vi "HandleStopSync.vi"(8 "error in (no error)":errorcluster, 11 "S4GUI in":refnum<class "S4GUI.lvclass">) -> (0 "error out":errorcluster, 3 "S4GUI out":refnum<class "S4GUI.lvclass">)   [LabVIEW 2018, in "S4GUI.lvclass"]
uses:
  S4GUI.lvclass
  S4GUI.lvclass/S4GUI.ctl
  Instrument/Instrument.lvclass/Instrument.ctl
  Instrument/Instrument.lvclass
  Device/Optics/Opt_Selector/Opt_Selector.lvclass
  Acquisition/Acquisition.lvclass
  StateMachine/State Machine.lvclass
  Channel/Channel.lvclass
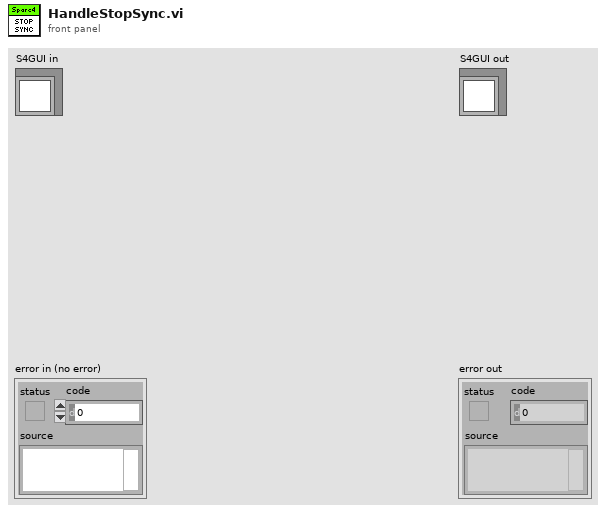
[diagram p1: front panel]
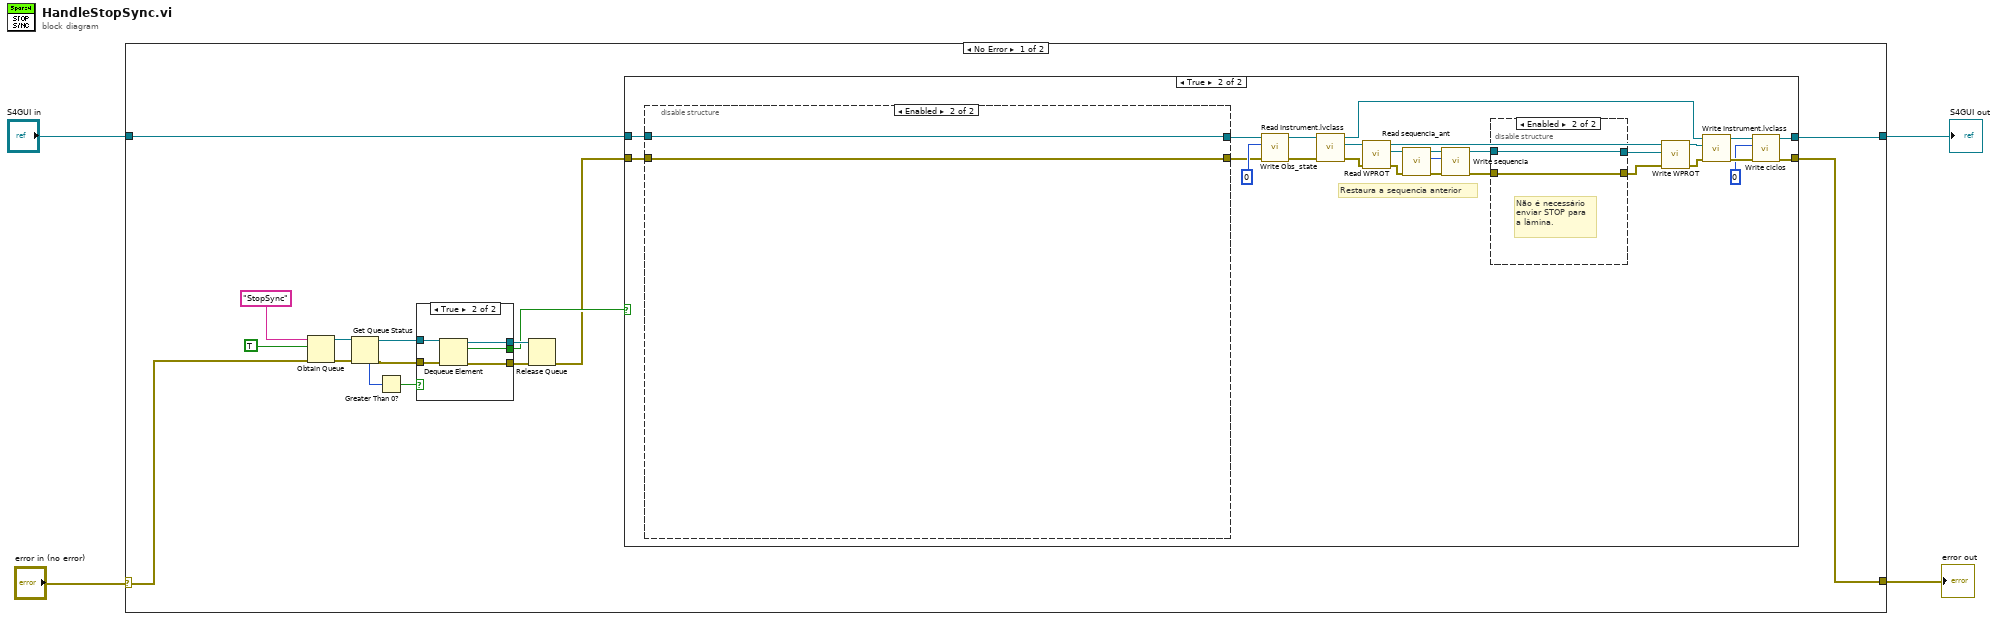
[diagram p0: block diagram]
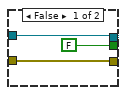
[diagram p2: hidden frame]
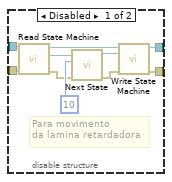
[diagram p4: hidden frame]
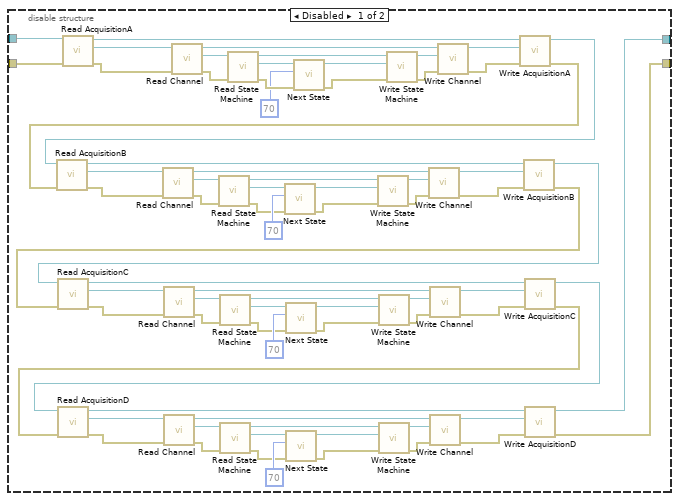
[diagram p5: hidden frame]
diagram:
  n1 = case shown="No Error" "error in (no error)" {
    selector: "error in (no error)" -> [w7 w147]
    tunnel: [w6 w147] -> w3
    tunnel: [w5 w146] -> w1
    tunnel: "S4GUI in" -> [w8 w146]
    frame No Error {
      n2 = Obtain Queue(name (unnamed)="StopSync", element data type=TRUE, error in (no error)=w7) -> (queue out=w17:refnum<queue>, error out=w18:errorcluster)  [unwired: 2 in, 1 out]
      n3 = Get Queue Status(queue=w17, error in (no error)=w18) -> (queue out=w14:refnum<queue>, error out=w13:errorcluster, # elements in queue=w16:i32)  [unwired: 1 in, 5 out]
      n4 = Greater Than 0?(x=w16) -> (x > 0?=w15:bool)
      n5 = case shown="True" w15 {
        tunnel: w14 -> [w22 w27]
        tunnel: w13 -> [w21 w28]
        tunnel: [FALSE w26] -> w10
        tunnel: [w22 w25] -> w12
        tunnel: [w21 w24] -> w11
        frame False {
        }
        frame True {
          n6 = Dequeue Element(queue=w27, error in (no error)=w28) -> (queue out=w25:refnum<queue>, element=w26:bool, error out=w24:errorcluster)  [unwired: 1 in, 1 out]
        }
      }
      n7 = Release Queue(queue=w12, error in (no error)=w11) -> (error out=w9:errorcluster)  [unwired: 1 in, 2 out]
      n8 = case shown="True" w10 {
        tunnel: w9 -> [w29 w54]
        tunnel: w8 -> [w30 w53]
        tunnel: [w29 w31] -> w6
        tunnel: [w30 w32] -> w5
        frame False {
        }
        frame True {
          # "Restaura a sequencia anterior"
          n9 = disable-structure shown="Enabled" {
            disable-tunnel: [w73 w145] -> w56
            disable-tunnel: [w72 w144] -> w55
            disable-tunnel: w54 -> [w71 w144]
            disable-tunnel: w53 -> [w70 w145]
            frame Disabled {
              n10 = call-dynamic "Read AcquisitionA.vi"("error in (no error)"=w71, "S4ACS_GUI in"=w70) -> ("error out"=w131:errorcluster, "Acquisition.lvclass"=w130:refnum<class "Acquisition.lvclass">, "S4ACS_GUI out"=w128:refnum<class "S4GUI.lvclass">)  [unwired: 7 in]
              n11 = call-dynamic "Read Channel.vi"("error in (no error)"=w131, "Acquisition in"=w130) -> ("error out"=w133:errorcluster, "Channel.lvclass"=w132:refnum<class "Channel.lvclass">, "Acquisition out"=w141:refnum<class "Acquisition.lvclass">)  [unwired: 7 in]
              n12 = call-dynamic "Read State Machine.vi"("error in (no error)"=w133, "Device in"=w132) -> ("error out"=w135:errorcluster, "State Machine.lvclass"=w134:refnum<class "State Machine.lvclass">, "Device out"=w137:refnum<class "Channel.lvclass">)  [unwired: 7 in]
              n13 = call "Next State.vi"("error in (no error)"=w135, "New_State"=u32 70, "State Machine in"=w134) -> ("error out"=w138:errorcluster, "State Machine out"=w136:refnum<class "State Machine.lvclass">)  [unwired: 7 in]
              n14 = call-dynamic "Write State Machine.vi"("error in (no error)"=w138, "State Machine.lvclass"=w136, "Device in"=w137) -> ("error out"=w142:errorcluster, "Device out"=w143:refnum<class "Channel.lvclass">)  [unwired: 7 in]
              n15 = call-dynamic "Write Channel.vi"("error in (no error)"=w142, "Channel.lvclass"=w143, "Acquisition in"=w141) -> ("error out"=w140:errorcluster, "Acquisition out"=w139:refnum<class "Acquisition.lvclass">)  [unwired: 7 in]
              n16 = call-dynamic "Write AcquisitionA.vi"("error in (no error)"=w140, "Acquisition.lvclass"=w139, "S4ACS_GUI in"=w128) -> ("error out"=w117:errorcluster, "S4ACS_GUI out"=w116:refnum<class "S4GUI.lvclass">)  [unwired: 7 in]
              n17 = call "Read AcquisitionB.vi"("error in (no error)"=w117, "S4ACS_GUI in"=w116) -> ("error out"=w110:errorcluster, "Acquisition.lvclass"=w114:refnum<class "Acquisition.lvclass">, "S4ACS_GUI out"=w115:refnum<class "S4GUI.lvclass">)  [unwired: 7 in]
              n18 = call-dynamic "Read Channel.vi"("error in (no error)"=w110, "Acquisition in"=w114) -> ("error out"=w125:errorcluster, "Channel.lvclass"=w126:refnum<class "Channel.lvclass">, "Acquisition out"=w112:refnum<class "Acquisition.lvclass">)  [unwired: 7 in]
              n19 = call-dynamic "Read State Machine.vi"("error in (no error)"=w125, "Device in"=w126) -> ("error out"=w123:errorcluster, "State Machine.lvclass"=w124:refnum<class "State Machine.lvclass">, "Device out"=w121:refnum<class "Channel.lvclass">)  [unwired: 7 in]
              n20 = call "Next State.vi"("error in (no error)"=w123, "New_State"=u32 70, "State Machine in"=w124) -> ("error out"=w120:errorcluster, "State Machine out"=w122:refnum<class "State Machine.lvclass">)  [unwired: 7 in]
              n21 = call-dynamic "Write State Machine.vi"("error in (no error)"=w120, "State Machine.lvclass"=w122, "Device in"=w121) -> ("error out"=w119:errorcluster, "Device out"=w118:refnum<class "Channel.lvclass">)  [unwired: 7 in]
              n22 = call-dynamic "Write Channel.vi"("error in (no error)"=w119, "Channel.lvclass"=w118, "Acquisition in"=w112) -> ("error out"=w111:errorcluster, "Acquisition out"=w113:refnum<class "Acquisition.lvclass">)  [unwired: 7 in]
              n23 = call "Write AcquisitionB.vi"("error in (no error)"=w111, "Acquisition.lvclass"=w113, "S4ACS_GUI in"=w115) -> ("error out"=w77:errorcluster, "S4ACS_GUI out"=w76:refnum<class "S4GUI.lvclass">)  [unwired: 7 in]
              n24 = call-dynamic "Read AcquisitionC.vi"("error in (no error)"=w77, "S4ACS_GUI in"=w76) -> ("error out"=w94:errorcluster, "Acquisition.lvclass"=w98:refnum<class "Acquisition.lvclass">, "S4ACS_GUI out"=w99:refnum<class "S4GUI.lvclass">)  [unwired: 7 in]
              n25 = call-dynamic "Read Channel.vi"("error in (no error)"=w94, "Acquisition in"=w98) -> ("error out"=w107:errorcluster, "Channel.lvclass"=w108:refnum<class "Channel.lvclass">, "Acquisition out"=w96:refnum<class "Acquisition.lvclass">)  [unwired: 7 in]
              n26 = call-dynamic "Read State Machine.vi"("error in (no error)"=w107, "Device in"=w108) -> ("error out"=w105:errorcluster, "State Machine.lvclass"=w106:refnum<class "State Machine.lvclass">, "Device out"=w103:refnum<class "Channel.lvclass">)  [unwired: 7 in]
              n27 = call "Next State.vi"("error in (no error)"=w105, "New_State"=u32 70, "State Machine in"=w106) -> ("error out"=w102:errorcluster, "State Machine out"=w104:refnum<class "State Machine.lvclass">)  [unwired: 7 in]
              n28 = call-dynamic "Write State Machine.vi"("error in (no error)"=w102, "State Machine.lvclass"=w104, "Device in"=w103) -> ("error out"=w101:errorcluster, "Device out"=w100:refnum<class "Channel.lvclass">)  [unwired: 7 in]
              n29 = call-dynamic "Write Channel.vi"("error in (no error)"=w101, "Channel.lvclass"=w100, "Acquisition in"=w96) -> ("error out"=w95:errorcluster, "Acquisition out"=w97:refnum<class "Acquisition.lvclass">)  [unwired: 7 in]
              n30 = call-dynamic "Write AcquisitionC.vi"("error in (no error)"=w95, "Acquisition.lvclass"=w97, "S4ACS_GUI in"=w99) -> ("error out"=w75:errorcluster, "S4ACS_GUI out"=w74:refnum<class "S4GUI.lvclass">)  [unwired: 7 in]
              n31 = call-dynamic "Read AcquisitionD.vi"("error in (no error)"=w75, "S4ACS_GUI in"=w74) -> ("error out"=w78:errorcluster, "Acquisition.lvclass"=w82:refnum<class "Acquisition.lvclass">, "S4ACS_GUI out"=w83:refnum<class "S4GUI.lvclass">)  [unwired: 7 in]
              n32 = call-dynamic "Read Channel.vi"("error in (no error)"=w78, "Acquisition in"=w82) -> ("error out"=w91:errorcluster, "Channel.lvclass"=w92:refnum<class "Channel.lvclass">, "Acquisition out"=w80:refnum<class "Acquisition.lvclass">)  [unwired: 7 in]
              n33 = call-dynamic "Read State Machine.vi"("error in (no error)"=w91, "Device in"=w92) -> ("error out"=w89:errorcluster, "State Machine.lvclass"=w90:refnum<class "State Machine.lvclass">, "Device out"=w87:refnum<class "Channel.lvclass">)  [unwired: 7 in]
              n34 = call "Next State.vi"("error in (no error)"=w89, "New_State"=u32 70, "State Machine in"=w90) -> ("error out"=w86:errorcluster, "State Machine out"=w88:refnum<class "State Machine.lvclass">)  [unwired: 7 in]
              n35 = call-dynamic "Write State Machine.vi"("error in (no error)"=w86, "State Machine.lvclass"=w88, "Device in"=w87) -> ("error out"=w85:errorcluster, "Device out"=w84:refnum<class "Channel.lvclass">)  [unwired: 7 in]
              n36 = call-dynamic "Write Channel.vi"("error in (no error)"=w85, "Channel.lvclass"=w84, "Acquisition in"=w80) -> ("error out"=w79:errorcluster, "Acquisition out"=w81:refnum<class "Acquisition.lvclass">)  [unwired: 7 in]
              n37 = call-dynamic "Write AcquisitionD.vi"("error in (no error)"=w79, "Acquisition.lvclass"=w81, "S4ACS_GUI in"=w83) -> ("error out"=w72:errorcluster, "S4ACS_GUI out"=w73:refnum<class "S4GUI.lvclass">)  [unwired: 7 in]
            }
            frame Enabled {
            }
          }
          n38 = call-dynamic "Write Obs_state.vi"("error in (no error)"=w55, "Obs_state"=u32 0, "S4ACS_GUI in"=w56) -> ("error out"=w33:errorcluster, "S4ACS_GUI out"=w34:refnum<class "S4GUI.lvclass">)  [unwired: 7 in]
          n39 = call "Read Instrument.lvclass.vi"("error in (no error)"=w33, "S4ACS_GUI in"=w34) -> ("error out"=w47:errorcluster, "Instrument.lvclass"=w49:refnum<class "Instrument.lvclass">, "S4ACS_GUI out"=w48:refnum<class "S4GUI.lvclass">)  [unwired: 7 in]
          n40 = call "Read WPROT.vi"("error in (no error)"=w47, "Instrument in"=w49) -> ("error out"=w42:errorcluster, "Opt_Selector.lvclass"=w45:refnum<class "Opt_Selector.lvclass">, "Instrument out"=w50:refnum<class "Instrument.lvclass">)  [unwired: 7 in]
          n41 = call-dynamic "Read sequencia_ant.vi"("error in (no error)"=w42, "Opt_Selector in"=w45) -> ("error out"=w41:errorcluster, "sequencia_ant"=w43:u16, "Opt_Selector out"=w44:refnum<class "Opt_Selector.lvclass">)  [unwired: 7 in]
          n42 = call-dynamic "Write sequencia.vi"("error in (no error)"=w41, "sequencia"=w43, "Opt_Selector in"=w44) -> ("error out"=w39:errorcluster, "Opt_Selector out"=w40:refnum<class "Opt_Selector.lvclass">)  [unwired: 7 in]
          n43 = disable-structure shown="Enabled" {
            disable-tunnel: w40 -> [w64 w69]
            disable-tunnel: w39 -> [w63 w68]
            disable-tunnel: [w59 w68] -> w38
            disable-tunnel: [w58 w69] -> w37
            frame Disabled {
              # "Para movimento \nda lamina retardadora"
              n44 = call-dynamic "Read State Machine.vi"("error in (no error)"=w63, "Device in"=w64) -> ("error out"=w66:errorcluster, "State Machine.lvclass"=w61:refnum<class "State Machine.lvclass">, "Device out"=w62:refnum<class "Opt_Selector.lvclass">)  [unwired: 7 in]
              n45 = call "Next State.vi"("error in (no error)"=w66, "New_State"=10, "State Machine in"=w61) -> ("error out"=w65:errorcluster, "State Machine out"=w60:refnum<class "State Machine.lvclass">)  [unwired: 7 in]
              n46 = call-dynamic "Write State Machine.vi"("error in (no error)"=w65, "State Machine.lvclass"=w60, "Device in"=w62) -> ("error out"=w59:errorcluster, "Device out"=w58:refnum<class "Opt_Selector.lvclass">)  [unwired: 7 in]
            }
            frame Enabled {
              # "Não é necessário\nenviar STOP para\na lâmina."
            }
          }
          n47 = call "Write WPROT.vi"("error in (no error)"=w38, "Opt_Selector.lvclass"=w37, "Instrument in"=w50) -> ("error out"=w35:errorcluster, "Instrument out"=w36:refnum<class "Instrument.lvclass">)  [unwired: 7 in]
          n48 = call "Write Instrument.lvclass.vi"("error in (no error)"=w35, "Instrument.lvclass"=w36, "S4ACS_GUI in"=w48) -> ("error out"=w51:errorcluster, "S4ACS_GUI out"=w52:refnum<class "S4GUI.lvclass">)  [unwired: 7 in]
          n49 = call-dynamic "Write ciclos.vi"("error in (no error)"=w51, "ciclos"=u32 0, "S4ACS_GUI in"=w52) -> ("error out"=w31:errorcluster, "S4ACS_GUI out"=w32:refnum<class "S4GUI.lvclass">)  [unwired: 7 in]
        }
      }
    }
    frame Error {
    }
  }
  "error out" <- w3
  "S4GUI out" <- w1
